vi "2021 Advent puzzle 02b.vi"() -> ()   [LabVIEW 2021]
panel:
  out "output 1":string
  out "64bit integer":i64
  out "X":i64
  out "Y":i64
  out "x*y":i64
  out "y":i64
  out "x":i64
  # "1451208"
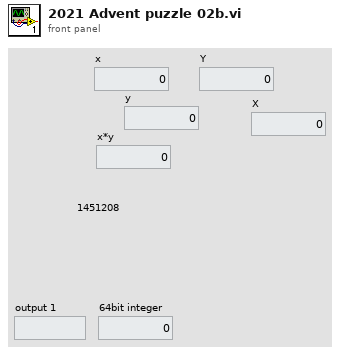
[diagram p1: front panel]
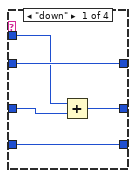
[diagram p2: hidden frame]
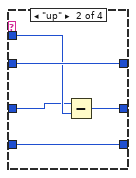
[diagram p3: hidden frame]
diagram:
  w2 = i64 0 ("index")
  (unwired) "forward 5\ndown 5\nforward 8\nup 3\ndown 8\nforward 2"
  # "find end position"
  n1 = Spreadsheet String To Array(delimiter (Tab)="\n", format string="", spreadsheet string="forward 9\ndown 3\ndown 8\nforward 2\nup 3\nforward 5\nup 8\ndown 2\ndown 5\nup 7\ndown 9\nforward 4\nup 5\ndown 9\nforward 2\nforward 2\nforward 8\ndown 6\nforward 2\nup 9\nup 5\ndown 2\nforward 5\ndown 8\nforward 3\nup 4\nforward 5\nforward 7\ndown 8\ndown 6\nup 7\ndown 3\nforward 4\nup 8\ndown 5\ndown 3\ndown 6\ndown 8\nforward 1\nforward 9\nforward 4\nup 7\ndown 4\nforward 7\nforward 3\nforward 9\ndown 1\ndown 3\nup 9\ndown 3\nforward 9\nup 6\nup 9\ndown 8\nup 3\ndown 1\nup 8\ndown 8\ndown 2\ndown 4\ndown 4\nup 3\ndown 6\ndown 1\ndown 3\nforward 1\nup 5\nforward 5\nforward 8\ndown 2\nforward 6\nforward 2\nup 7\nforward 6\ndown 8\nforward 6\nforward 5\nup 9\nforward 5\nup 5\nforward 9\ndown 2\ndown 4\ndown 3\ndown 8\nforward 9\nforward 6\nforward 2\nup 7\ndown 7\nup 3\nforward 4\nforward 5\ndown 7\nforward 5\nup 9\nforward 6\nforward 6\nforward 1\ndown 6\nforward 9\nup 2\ndown 7\ndown 8\ndown 6\nup 5\ndown 8\ndown 8\nforward 7\ndown 6\nup 5\ndown 9\ndown 3\nforward 2\ndown 4\nforward 8\ndown 5\nup 5\nforward 7\nup 2\nup 2\ndown 4\nforward 4\ndown 5\nup 8\ndown 2\nforward 4\ndown 9\nforward 8\ndown 5\ndown 6\ndown 7\nup 7\nup 5\nup 7\nforward 7\nforward 8\ndown 2\nforward 3\ndown 2\ndown 7\ndown 4\ndown 2\nforward 3\nforward 5\ndown 3\ndown 7\nup 7\ndown 7\nup 5\nforward 1\ndown 8\ndown 2\nup 4\nup 5\ndown 8\nforward 9\ndown 3\ndown 9\nforward 8\nforward 1\nforward 1\ndown 2\nup 9\ndown 2\nup 8\ndown 6\nup 8\nforward 7\ndown 5\nforward 7\ndown 8\nforward 8\ndown 7\nup 9\nup 2\nup 6\ndown 5\ndown 9\nforward 2\nup 3\ndown 4\nup 5\nup 4\ndown 9\nforward 7\nforward 7\ndown 3\nforward 4\nforward 9\nup 8\nforward 3\ndown 1\nforward 2\ndown 7\ndown 3\ndown 7\ndown 7\nforward 8\nforward 4\nforward 7\nup 1\ndown 4\nup 9\ndown 2\ndown 1\nforward 6\ndown 3\nforward 7\nforward 8\nup 9\nup 2\nup 2\nforward 7\nup 2\nup 5\nforward 5\ndown 3\nforward 8\nforward 1\nup 4\ndown 6\ndown 5\nforward 4\nup 9\nforward 8\nup 4\ndown 8\ndown 3\ndown 3\ndown 7\nforward 2\nforward 4\ndown 9\ndown 7\ndown 2\nup 3\nup 3\nforward 8\nforward 7\nforward 8\ndown 5\nup 5\nforward 3\nforward 6\nup 7\nup 1\nforward 2\nforward 5\ndown 5\nforward 8\ndown 2\ndown 4\nforward 2\ndown 7\ndown 3\ndown 5\nforward 9\ndown 7\ndown 8\nup 1\nup 2\ndown 8\nforward 7\nforward 8\ndown 8\nforward 5\nup 7\nforward 3\nup 2\ndown 7\nforward 1\ndown 2\nup 7\nup 4\ndown 2\nforward 1\nup 5\nforward 2\nup 2\nforward 3\nforward 9\nforward 2\nforward 8\nforward 2\nup 7\ndown 8\ndown 7\nforward 2\nforward 7\ndown 1\nforward 2\nup 1\nup 6\ndown 3\ndown 6\nforward 7\ndown 4\nforward 5\nforward 6\nup 3\nforward 3\ndown 6\nforward 8\nup 8\nforward 4\ndown 3\nforward 3\ndown 4\ndown 7\nforward 9\nforward 2\nup 2\nforward 8\ndown 6\nforward 6\ndown 9\ndown 9\nforward 8\ndown 1\nforward 9\ndown 1\ndown 6\ndown 8\ndown 5\ndown 5\nforward 3\nforward 3\ndown 2\ndown 5\nforward 9\ndown 2\ndown 8\ndown 3\nforward 9\nup 2\ndown 4\ndown 9\nforward 9\nforward 1\nforward 5\nup 9\ndown 1\ndown 6\nforward 6\nforward 5\nforward 8\ndown 2\nforward 8\ndown 4\ndown 2\ndown 6\ndown 6\nup 3\nup 8\nforward 1\ndown 1\nup 8\ndown 3\ndown 4\nup 9\nup 1\ndown 7\ndown 7\nup 1\nup 2\nforward 5\nup 8\nforward 2\ndown 3\nforward 1\nup 5\nforward 6\nforward 2\ndown 6\nup 2\nforward 2\nforward 1\ndown 3\nforward 4\nup 8\nforward 5\ndown 4\nforward 2\ndown 8\ndown 7\nup 7\ndown 8\nforward 1\ndown 4\nup 9\ndown 6\nup 6\nup 6\ndown 2\nforward 1\nforward 8\ndown 6\nup 3\ndown 7\nforward 9\nup 1\nup 4\nforward 7\ndown 7\nforward 1\ndown 6\ndown 4\ndown 7\ndown 8\ndown 8\nforward 4\ndown 6\ndown 6\ndown 5\nforward 6\nup 9\nup 3\ndown 4\nforward 8\ndown 7\nforward 6\nup 3\nforward 1\nforward 1\ndown 8\nforward 7\nforward 4\nforward 6\nup 1\nforward 7\nup 8\nforward 2\nforward 6\nforward 8\ndown 9\ndown 8\nup 9\nup 4\nup 2\nforward 2\nforward 8\nup 2\nforward 3\nforward 2\nup 2\nup 5\nup 8\nforward 4\nforward 8\nforward 3\nup 5\ndown 1\nforward 2\ndown 7\ndown 8\nforward 3\nup 1\nforward 5\nforward 7\nforward 9\nup 7\nforward 4\ndown 4\nup 2\nforward 4\nforward 5\nforward 3\nup 9\nforward 6\nforward 8\ndown 9\ndown 1\nforward 1\ndown 5\ndown 2\nforward 9\ndown 2\nup 9\ndown 1\nforward 5\nforward 8\nup 2\nforward 6\ndown 4\ndown 9\nforward 4\nforward 1\ndown 3\ndown 3\nup 5\nforward 5\ndown 6\nforward 3\ndown 2\nforward 8\ndown 7\ndown 2\ndown 1\nforward 2\nup 5\nforward 9\nforward 3\nforward 5\ndown 4\nup 7\nforward 6\ndown 3\nforward 1\nforward 7\nforward 1\nup 4\ndown 2\ndown 7\nup 9\nforward 9\ndown 8\ndown 1\nup 2\ndown 3\nforward 7\ndown 8\ndown 5\ndown 5\nup 8\nforward 1\ndown 5\nforward 8\nup 7\ndown 1\nforward 9\ndown 4\nforward 8\nforward 5\nforward 7\nforward 8\nforward 3\nup 9\nforward 3\ndown 7\ndown 5\nup 8\nforward 3\nup 6\nforward 8\nup 3\ndown 5\nforward 5\nforward 6\nforward 4\nforward 3\nforward 8\nup 9\nforward 2\ndown 6\ndown 4\ndown 5\nforward 7\ndown 2\nup 5\nforward 2\nforward 5\ndown 9\nforward 8\ndown 8\nforward 6\ndown 9\ndown 7\nup 9\nforward 3\nforward 3\nup 5\ndown 2\nforward 5\ndown 6\ndown 6\ndown 2\ndown 3\ndown 4\nforward 7\nup 1\ndown 7\nforward 7\nup 1\nforward 3\nup 6\ndown 7\ndown 5\nforward 9\nforward 2\ndown 5\nforward 9\ndown 5\nforward 9\nforward 1\ndown 4\nforward 9\ndown 5\nforward 8\ndown 6\ndown 4\ndown 5\nforward 9\ndown 1\nforward 6\nforward 9\ndown 1\ndown 1\nup 2\nforward 5\nforward 3\ndown 4\nup 8\nforward 8\ndown 2\nforward 3\nforward 1\ndown 7\nforward 6\nforward 5\nup 7\nup 8\ndown 5\nup 3\ndown 8\nforward 6\nforward 5\nforward 6\nup 1\nup 8\nup 7\ndown 5\nforward 3\nforward 9\nup 9\nup 4\nup 7\nup 8\nforward 7\nforward 3\nforward 9\ndown 7\nforward 3\ndown 6\nforward 9\ndown 1\nforward 3\ndown 1\nforward 8\nforward 7\ndown 2\nforward 1\nforward 6\nforward 7\ndown 3\ndown 2\ndown 1\nforward 7\nforward 4\ndown 6\nup 4\nforward 4\nforward 9\nforward 3\ndown 1\nup 2\ndown 3\ndown 5\nforward 7\nforward 5\nup 1\ndown 2\ndown 3\ndown 8\nforward 1\ndown 4\nforward 5\ndown 5\nup 6\ndown 6\ndown 8\nforward 1\nforward 9\nup 5\nforward 2\ndown 9\ndown 5\ndown 1\ndown 4\ndown 9\ndown 8\nforward 2\nforward 4\nup 2\nforward 3\ndown 8\ndown 5\nup 5\nforward 8\nup 2\ndown 8\nup 3\nforward 7\ndown 7\nforward 8\ndown 7\ndown 3\nup 6\nforward 5\nup 4\nup 5\nforward 9\nforward 6\ndown 9\nforward 5\ndown 5\ndown 3\nforward 2\ndown 1\nup 9\nup 8\ndown 6\ndown 1\nforward 9\nforward 4\nforward 2\nup 1\nforward 5\nforward 9\nup 5\nforward 8\nforward 4\ndown 4\ndown 4\ndown 2\nforward 1\nforward 7\ndown 9\nforward 4\ndown 5\ndown 4\ndown 7\ndown 2\nforward 9\ndown 3\nforward 6\nforward 3\ndown 9\ndown 3\ndown 4\ndown 9\ndown 9\nup 6\ndown 5\nup 4\ndown 1\ndown 1\nforward 9\nforward 7\ndown 9\nforward 4\ndown 8\ndown 7\nforward 7\nforward 4\nup 2\nup 5\nforward 2\nforward 7\ndown 1\nforward 6\nforward 6\nforward 3\nforward 8\ndown 2\nup 2\nforward 7\nup 5\ndown 1\ndown 5\nforward 8\ndown 6\nforward 8\ndown 5\ndown 4\ndown 6\nforward 5\ndown 1\nforward 9\nforward 8\nup 5\ndown 6\nforward 5\nup 5\ndown 4\nforward 1\ndown 2\ndown 5\ndown 3\nforward 2\ndown 9\nforward 1\nforward 1\nforward 1\nforward 8\nforward 2\ndown 8\ndown 6\nup 1\nforward 6\ndown 3\ndown 4\nup 9\ndown 3\ndown 3\nup 7\ndown 4\nforward 4\nforward 9\ndown 3\ndown 8\nforward 5\ndown 3\ndown 6\ndown 7\nforward 1\nup 2\nforward 8\ndown 1\ndown 4\nup 9\nforward 9\nup 4\nup 2\nforward 3\nforward 4\ndown 2\ndown 2\ndown 6\nforward 6\nforward 8\ndown 6\nup 6\ndown 5\nforward 1\ndown 4\nup 9\nforward 1\nforward 3\ndown 1\ndown 4\nup 6\nforward 5\nforward 6\nup 9\nup 9\ndown 2\nup 6\nforward 1\nforward 2\nforward 3\nforward 3\nforward 6\nup 2\ndown 8\ndown 9\nforward 7\nup 1\nup 3\ndown 2\nforward 3\ndown 8\nforward 9\ndown 3\nforward 6\nup 2\nforward 7\ndown 2\nforward 5\ndown 4\ndown 2\nup 8\nforward 3\nforward 5\nforward 9\nforward 5\nforward 3\nup 9\ndown 7\nforward 4\nforward 2\nforward 7\ndown 5\nup 6\nup 6\nforward 8\ndown 2\nforward 1\nup 1\nup 9\nup 8\nup 3\nup 4\ndown 2\nup 7\ndown 4\nup 5\ndown 1\nup 9\ndown 5\ndown 9\ndown 4\nup 2\ndown 8\nup 2\nup 7\nup 9\nforward 4\nforward 2\nforward 1\nforward 6\nforward 8\nup 5\nforward 5\nforward 5\ndown 4\nup 6\nforward 3\ndown 9\ndown 7\nforward 4\ndown 3\nup 1\nforward 4\ndown 2\ndown 6\nup 3\nup 1\ndown 9\ndown 7\ndown 9\nforward 3\nforward 8\ndown 8\nup 7\nup 6\ndown 2\ndown 9\ndown 1\ndown 9\nforward 6\nup 4\ndown 3\nforward 5\nup 3\nup 9\nup 8\nforward 6\ndown 8\nforward 6\nforward 6\nforward 5\nup 4\ndown 4\nup 6\nup 4\nforward 2\ndown 5\nforward 9\nup 7\nup 6\ndown 4\nforward 7\nforward 6\nup 2\ndown 8\ndown 6\nforward 5\nup 2\nforward 5\nforward 1\nup 9\ndown 8\nforward 7\nup 4\nforward 8\ndown 4\nforward 3\nforward 3\ndown 9\nforward 4\nforward 9\nup 8\nforward 7\nforward 3\nforward 9\nforward 4\nup 3\nforward 2\nforward 7", array type (2D Dbl)=string[] []) -> (array=w6:string[])
  n2 = for {
    tunnel: w6 -> [w21] mode=indexing
    shift-right: [w15] -> w5
    shift-left: w2 -> [w17]
    shift-right: [w14] -> _
    shift-left: w2 -> [w16]
    tunnel: [w12] -> _
    shift-right: [w10] -> w1
    shift-left: w2 -> [w11]
    i -> [w12]
    # "aim"
    # "depth"
    # "x"
    n3 = Scan From String(format string="%s %d", input string=w21) -> (output 1=w19:string, output 2=w18:i32)  [unwired: 4 in, 3 out]
    "output 1" <- w19
    n4 = To Quad Integer(1:w18) -> (0:w13:i64)
    "64bit integer" <- w13
    n5 = case shown="\"forward\"" w19 {
      tunnel: w13 -> [w23 w30 _ w38]
      tunnel: w17 -> [w26 w31 w34 w41]
      tunnel: w16 -> [w25 w28 w33 w37]
      tunnel: [w26 w31 w34 w40] -> w15
      tunnel: [w24 w29 w33 w37] -> w14
      tunnel: [w22 w27 w32 w36] -> w10
      tunnel: w11 -> [w22 w27 w32 w39]
      frame "down" {
        n6 = Add(x=w23, y=w25) -> (x+y=w24:i64)
      }
      frame "up" {
        n7 = Subtract(x=w28, y=w30) -> (x-y=w29:i64)
      }
      frame Default {
      }
      frame "forward" {
        n8 = Multiply(x=w37, y=w38) -> (x*y=w35:i64)
        n9 = Add(x=w38, y=w41) -> (x+y=w40:i64)
        n10 = Add(x=w35, y=w39) -> (x+y=w36:i64)
      }
    }
    "Y" <- w14
    "X" <- w15
  }
  "x" <- w5
  "y" <- w1
  n11 = Multiply(x=w5, y=w1) -> (x*y=→"x*y":i64)
